vi "Execute Logging Command.vi"(8 "error in (no error)":errorcluster, 10 "command":T1={"Command"=enum."Log Plugin State", "Parameters"={"arg1"=0, "arg2"=0}}, 11 "Logging Thread in":refnum<class "Logging Thread.lvclass">) -> (0 "error out":errorcluster, 3 "Logging Thread out":refnum<class "Logging Thread.lvclass">)   [LabVIEW 2017, in "DSF Core.lvlib" / "Logging Thread.lvclass"]
uses:
  Logging Thread.lvclass
  C:/Git/niveristand-data-sharing-framework-custom-device/Core/Classes/Thread/Thread.lvclass
  Interface/Logging/Command Data.ctl
  Interface/Logging/Command.ctl
  Interface/Logging/Parameters.ctl
  Logging Thread.lvclass/Logging Thread.ctl
  Interface/Logging/Response Data.ctl
  Interface/Logging/Response.ctl
  Interface/Logging/Framework State Parameters.ctl
  Framework/Framework States.ctl
  Pointers/Error/Error Sizes.ctl
  Interface/Logging/Plugin State Parameters.ctl
  Interface/Plugin/Command.ctl
  Interface/Logging/Dispatcher State Parameters.ctl
  Interface/Dispatcher/Command.ctl
  Interface/Logging/Send Logging Response.vi
  Thread.lvclass
  Interface/Logging/Logging Interface.lvclass
  Framework/Framework.lvclass
  Interface/Plugin/Plugin Interface.lvclass
  Pointers/Error/Error Pointer.lvclass
  Interface/Dispatcher/Dispatcher Interface.lvclass
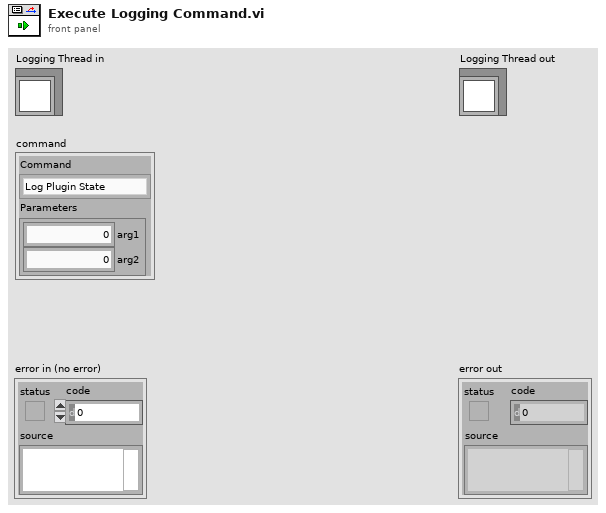
[diagram p1: front panel]
types:
  T1 = typedef "DSF Core.lvlib/Logging Interface.lvclass/Command Data.ctl" = cluster{"Command":T2, "Parameters":T3}
  T2 = typedef "DSF Core.lvlib/Logging Interface.lvclass/Command.ctl" = enum8{"Idle", "Start", "Log Framework State", "Log Plugin State", "Log Dispatcher State", "Shutdown"}
  T3 = typedef "DSF Core.lvlib/Logging Interface.lvclass/Parameters.ctl" = cluster{"arg1":u64, "arg2":u64}
  T4 = typedef "DSF Core.lvlib/Logging Interface.lvclass/Response Data.ctl" = cluster{"Response":T5, "Parameters":T3}
  T5 = typedef "DSF Core.lvlib/Logging Interface.lvclass/Response.ctl" = enum8{"General Ack", "Error", "Shutting Down"}
  T6 = typedef "DSF Core.lvlib/Error Pointer.lvclass/Error Sizes.ctl" = enum8{"256", "512", "1024"}
  T7 = typedef "DSF Core.lvlib/Logging Interface.lvclass/Framework State Parameters.ctl" = cluster{"state":T8, "unused":u8, "unused 2":u16, "unused 3":u32, "error pointer":u64}
  T8 = typedef "DSF Core.lvlib/Framework.lvclass/Framework States.ctl" = enum8{"Uninitialized", "Initialized", "Start", "Rx", "Tx", "Shutdown"}
  T9 = typedef "DSF Core.lvlib/Logging Interface.lvclass/Plugin State Parameters.ctl" = cluster{"state":T10, "Plugin ID":u8, "Thread ID":u8, "unused 0":u8, "unused 1":i32, "error pointer":u64}
  T10 = typedef "DSF Core.lvlib/Plugin Interface.lvclass/Command.ctl" = enum8{"Idle", "Start", "Set Inline Buffer", "Rx", "Tx", "Shutdown", "Error"}
  T11 = typedef "DSF Core.lvlib/Logging Interface.lvclass/Dispatcher State Parameters.ctl" = cluster{"state":T12, "unused":u8, "unused 2":u16, "unused 3":u32, "error pointer":u64}
  T12 = typedef "DSF Core.lvlib/Dispatcher Interface.lvclass/Command.ctl" = enum8{"Idle", "Start", "Rx", "Tx", "Set Inline Buffer", "Shutdown", "Error"}
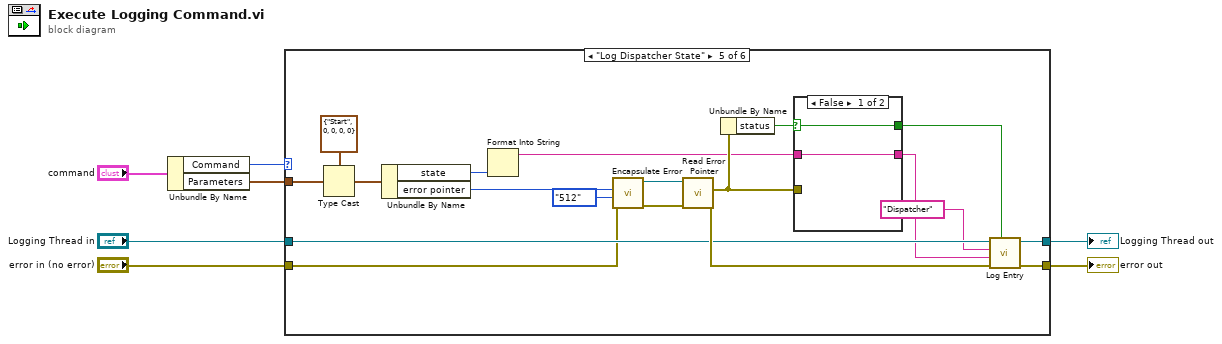
[diagram p0: block diagram]
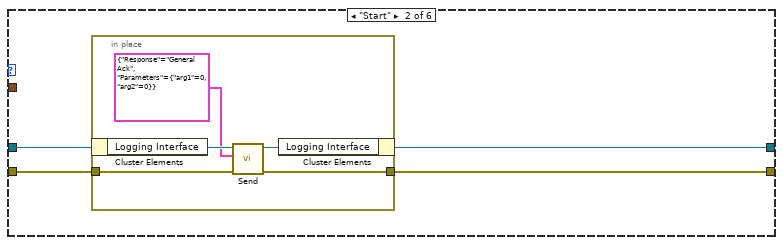
[diagram p3: hidden frame]
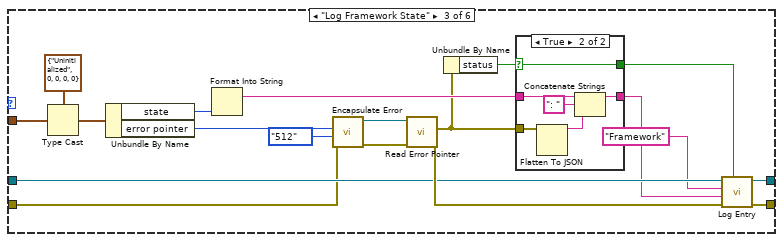
[diagram p4: hidden frame]
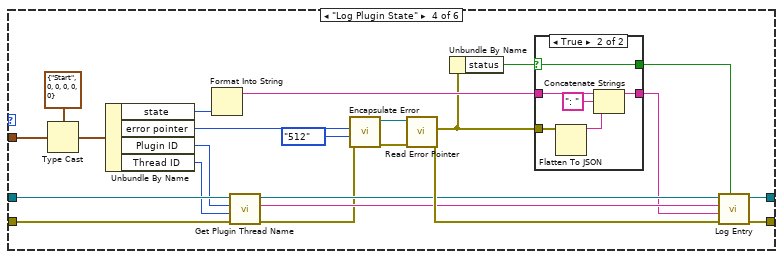
[diagram p6: hidden frame]
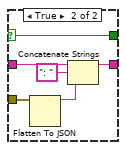
[diagram p8: hidden frame]
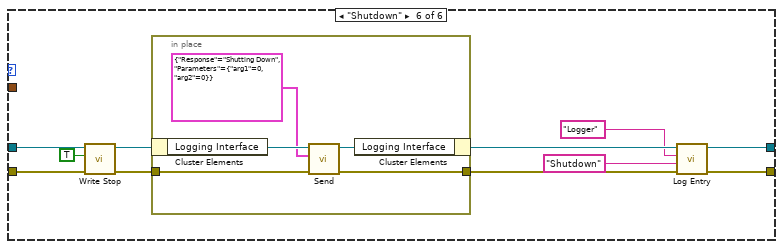
[diagram p9: hidden frame]
diagram:
  n1 = Unbundle By Name("command") -> ("Command"=w6:T2, "Parameters"=w5:T3)
  n2 = case shown="\"Log Dispatcher State\"" w6 {
    tunnel: w5 -> [_ _ w37 w68 w95 _]
    tunnel: "Logging Thread in" -> [w9 w13 w30 w61 w88 w113]
    tunnel: [w9 w10 w32 w63 w90 w106] -> w4
    tunnel: "error in (no error)" -> [w8 w12 w20 w60 w78 w114]
    tunnel: [w8 w11 w33 w64 w91 w107] -> w3
    frame "Idle" {
    }
    frame "Start" {
      n3 = in-place {
        in-place-border: w12 -> [w16]
        in-place-border: [w15] -> w11
        n4 = in-place-cluster #1(w13) -> ("Logging Interface"=w18:refnum<class "Logging Interface.lvclass">)
        n5 = call-poly "Send.vi"("error in (no error)"=w16, "response"=T4 {"Response"=enum."General Ack", "Parameters"={"arg1"=0, "arg2"=0}}, "Logging Interface in"=w18) -> ("error out"=w15:errorcluster, "Logging Interface out"=w17:refnum<class "Logging Interface.lvclass">)  [unwired: 7 in]
        n6 = in-place-cluster #1("Logging Interface"=w17) -> (w10:refnum<class "Logging Thread.lvclass">)
      }
    }
    frame "Log Framework State" {
      n7 = Type Cast(type=T7 {"state"=enum."Uninitialized", "unused"=0, "unused 2"=0, "unused 3"=0, "error pointer"=0} ("Parameters"), x=w37) -> (*(type *) &x=w35:T7)
      n8 = Unbundle By Name(w35) -> ("state"=w34:T8, "error pointer"=w19:u64)
      n9 = Format Into String(w34) -> (resulting string=w29:string)  [unwired: 3 in, 1 out]
      n10 = call "Encapsulate Error.vi"("error in (no error)"=w20, "error size"=Error_Sizes."512", "address"=w19) -> ("error out"=w22:errorcluster, "Error Pointer out"=w21:refnum<class "Error Pointer.lvclass">)  [unwired: 7 in]
      n11 = call "Read Error Pointer.vi"("error in"=w22, "Error Pointer in"=w21) -> ("error out"=w31:errorcluster, "error"=w26:errorcluster)  [unwired: 7 in, 1 out]
      n12 = Unbundle By Name(w26) -> ("status"=w25:bool)
      n13 = case shown="True" w25 {
        selector: w25 -> [w38 w41]
        tunnel: w29 -> [w39 w40]
        tunnel: [w39 w43] -> w28
        tunnel: w26 -> [_ w42]
        tunnel: [w38 w41] -> w24
        frame False {
        }
        frame True {
          n14 = Flatten To JSON(anything=w42) -> (JSON string=w44:string)  [unwired: 2 in, 1 out]
          n15 = Concatenate Strings(w40, ": " ("string"), w44) -> (w43:string)
        }
      }
      n16 = call "Log Entry.vi"("error? (F)"=w24, "error in (no error)"=w31, "line text"=w28, "line tag"="Framework", "Logging Thread in"=w30) -> ("error out"=w33:errorcluster, "Logging Thread out"=w32:refnum<class "Logging Thread.lvclass">)  [unwired: 5 in]
    }
    frame "Log Plugin State" {
      n17 = Type Cast(type=T9 {"state"=enum."Start", "Plugin ID"=0, "Thread ID"=0, "unused 0"=0, "unused 1"=0, "error pointer"=0} ("Parameters"), x=w68) -> (*(type *) &x=w66:T9)
      n18 = Unbundle By Name(w66) -> ("state"=w65:T10, "error pointer"=w47:u64, "Plugin ID"=w58:u8, "Thread ID"=w59:u8)
      n19 = Format Into String(w65) -> (resulting string=w55:string)  [unwired: 3 in, 1 out]
      n20 = call "Get Plugin Thread Name.vi"("error in (no error)"=w60, "Thread ID"=w59, "Plugin ID"=w58, "Logging Thread in"=w61) -> ("error out"=w50:errorcluster, "thread name"=w56:string, "Logging Thread out"=w57:refnum<class "Logging Thread.lvclass">)  [unwired: 5 in]
      n21 = call "Encapsulate Error.vi"("error in (no error)"=w50, "error size"=Error_Sizes."512", "address"=w47) -> ("error out"=w49:errorcluster, "Error Pointer out"=w48:refnum<class "Error Pointer.lvclass">)  [unwired: 7 in]
      n22 = call "Read Error Pointer.vi"("error in"=w49, "Error Pointer in"=w48) -> ("error out"=w62:errorcluster, "error"=w52:errorcluster)  [unwired: 7 in, 1 out]
      n23 = Unbundle By Name(w52) -> ("status"=w54:bool)
      n24 = case shown="True" w54 {
        selector: w54 -> [w69 w72]
        tunnel: w55 -> [w70 w71]
        tunnel: [w70 w74] -> w51
        tunnel: w52 -> [_ w73]
        tunnel: [w69 w72] -> w53
        frame False {
        }
        frame True {
          n25 = Flatten To JSON(anything=w73) -> (JSON string=w75:string)  [unwired: 2 in, 1 out]
          n26 = Concatenate Strings(w71, ": " ("string"), w75) -> (w74:string)
        }
      }
      n27 = call "Log Entry.vi"("error? (F)"=w53, "error in (no error)"=w62, "line text"=w51, "line tag"=w56, "Logging Thread in"=w57) -> ("error out"=w64:errorcluster, "Logging Thread out"=w63:refnum<class "Logging Thread.lvclass">)  [unwired: 5 in]
    }
    frame "Log Dispatcher State" {
      n28 = Type Cast(type=T11 {"state"=enum."Start", "unused"=0, "unused 2"=0, "unused 3"=0, "error pointer"=0} ("Parameters"), x=w95) -> (*(type *) &x=w93:T11)
      n29 = Unbundle By Name(w93) -> ("state"=w92:T12, "error pointer"=w77:u64)
      n30 = Format Into String(w92) -> (resulting string=w80:string)  [unwired: 3 in, 1 out]
      n31 = call "Encapsulate Error.vi"("error in (no error)"=w78, "error size"=Error_Sizes."512", "address"=w77) -> ("error out"=w79:errorcluster, "Error Pointer out"=w81:refnum<class "Error Pointer.lvclass">)  [unwired: 7 in]
      n32 = call "Read Error Pointer.vi"("error in"=w79, "Error Pointer in"=w81) -> ("error out"=w89:errorcluster, "error"=w85:errorcluster)  [unwired: 7 in, 1 out]
      n33 = Unbundle By Name(w85) -> ("status"=w86:bool)
      n34 = case shown="False" w86 {
        selector: w86 -> [w96 w99]
        tunnel: w80 -> [w97 w98]
        tunnel: [w97 w101] -> w84
        tunnel: w85 -> [_ w100]
        tunnel: [w96 w99] -> w83
        frame False {
        }
        frame True {
          n35 = Flatten To JSON(anything=w100) -> (JSON string=w102:string)  [unwired: 2 in, 1 out]
          n36 = Concatenate Strings(w98, ": " ("string"), w102) -> (w101:string)
        }
      }
      n37 = call "Log Entry.vi"("error? (F)"=w83, "error in (no error)"=w89, "line text"=w84, "line tag"="Dispatcher", "Logging Thread in"=w88) -> ("error out"=w91:errorcluster, "Logging Thread out"=w90:refnum<class "Logging Thread.lvclass">)  [unwired: 5 in]
    }
    frame "Shutdown" {
      n38 = call "Write Stop.vi"("error in (no error)"=w114, "stop"=TRUE, "Thread in"=w113) -> ("error out"=w111:errorcluster, "Thread out"=w110:refnum<class "Logging Thread.lvclass">)  [unwired: 7 in]
      n39 = in-place {
        in-place-border: w111 -> [w117]
        in-place-border: [w116] -> w108
        n40 = in-place-cluster #2(w110) -> ("Logging Interface"=w119:refnum<class "Logging Interface.lvclass">)
        n41 = call-poly "Send.vi"("error in (no error)"=w117, "response"=T4 {"Response"=enum."Shutting Down", "Parameters"={"arg1"=0, "arg2"=0}}, "Logging Interface in"=w119) -> ("error out"=w116:errorcluster, "Logging Interface out"=w118:refnum<class "Logging Interface.lvclass">)  [unwired: 7 in]
        n42 = in-place-cluster #2("Logging Interface"=w118) -> (w105:refnum<class "Logging Thread.lvclass">)
      }
      n43 = call "Log Entry.vi"("error in (no error)"=w108, "line text"="Shutdown", "line tag"="Logger", "Logging Thread in"=w105) -> ("error out"=w107:errorcluster, "Logging Thread out"=w106:refnum<class "Logging Thread.lvclass">)  [unwired: 6 in]
    }
  }
  "error out" <- w3
  "Logging Thread out" <- w4
